vi "Test_PicoScope_v2.vi"() -> ()   [LabVIEW 2015]
uses:
  Controls/PicoScope/pico_control_panel.ctl
  Controls/PicoScope/pico_channel_settings.ctl
  Controls/PicoScope/pico_trigger.ctl
  Controls/PicoScope/pico_init_settings.ctl
panel:
  out "Pico Scope Channel B":T1(graph)
  out "Pico Scope Channel A":T1(graph)
  in  "error in (no error)":errorcluster
  out "error out":errorcluster
  in  "PicoScope Acquisition Settings Input":T2={"Channel A Settings"={"Enabled"=TRUE, "Coupling"=1, "Range"=6, "Analogue Offset"=0.0}, "Channel B Settings"={"Enabled"=TRUE, "Coupling"=1, "Range"=6, "Analogue Offset"=0.0}, "Trigger Options"={"Trigger Enabled"=FALSE, "Trigger Source"=enum."Channel A", "Trigger Threshold (-5 to 5 V)"=0.0, "Trigger Slope"=2, "Trigger Delay (ms)"=0.0, "Auto Trigger Time (ms)"=1000}, "Pico Scope Inititalization Settings"={"USB Power"=FALSE, "Use Serial Number"=FALSE, "Resolution"=0, "Serial Number"="", "Handle"=0}, "Use PicoScope?"=FALSE, "Acquisition Settings"={"Pre Trigger Time (s)"=512.0, "Post Trigger Time (s)"=512.0, "Resolution (s)"=34.36, "Four Channel Device"=FALSE, "Number of Captures"=1.0}} {"Acquisition Settings"."Number of Captures" min=1.0 step=1.0; "Acquisition Settings"."Resolution (s)" min=1e-09 max=34.36 step=1e-09 format="%#_6p"; "Acquisition Settings"."Post Trigger Time (s)" min=0.0 format="%#_6p"; "Acquisition Settings"."Pre Trigger Time (s)" min=0.0 format="%#_6p"; "Pico Scope Inititalization Settings"."Resolution" items=["8-bit", "12-bit", "14-bit", "15-bit (max. 2 ch.)", "16-bit (max. 1 ch.)"]; "Trigger Options"."Trigger Slope" items=["Rising"=2, "Falling"=3]; "Channel B Settings"."Range" items=["10 mV", "20 mV", "50 mV", "100 mV", "200 mV", "500 mV", "1 V", "2 V", "5 V", "10 V", "20 V", "50 V ", "100 V"]; "Channel B Settings"."Coupling" items=["AC", "DC"]; "Channel A Settings"."Range" items=["10 mV", "20 mV", "50 mV", "100 mV", "200 mV", "500 mV", "1 V", "2 V", "5 V", "10 V", "20 V", "50 V ", "100 V"]; "Channel A Settings"."Coupling" items=["AC", "DC"]}
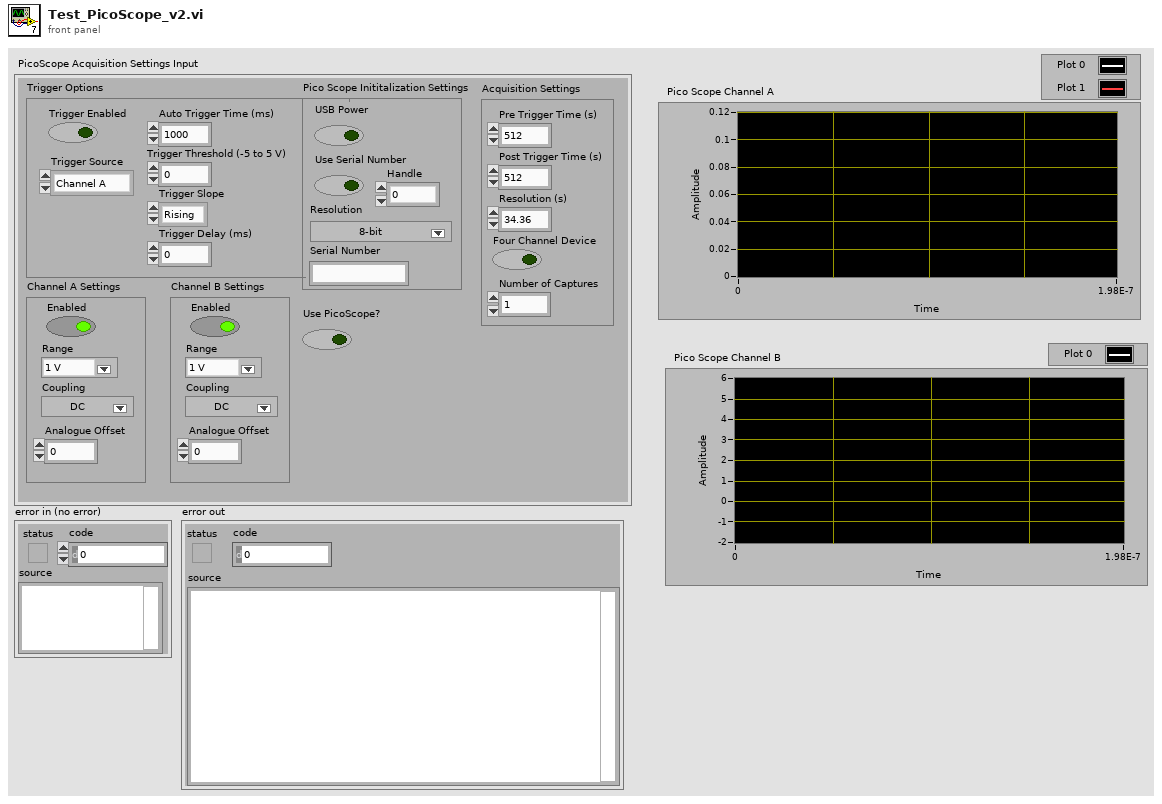
[diagram p1: front panel]
types:
  T1 = cluster{"Channel A Out":dbl[], "Channel A Out":dbl[]}[]
  T2 = typedef "pico_control_panel.ctl" = cluster{"Channel A Settings":T3, "Channel B Settings":T3, "Trigger Options":T4, "Pico Scope Inititalization Settings":T5, "Use PicoScope?":bool, "Acquisition Settings":cluster{"Pre Trigger Time (s)":dbl, "Post Trigger Time (s)":dbl, "Resolution (s)":dbl, "Four Channel Device":bool, "Number of Captures":dbl}}
  T3 = typedef "pico_channel_settings.ctl" = cluster{"Enabled":bool, "Coupling":i16, "Range":u16, "Analogue Offset":sgl}
  T4 = typedef "pico_trigger.ctl" = cluster{"Trigger Enabled":bool, "Trigger Source":enum16{"Channel A", "Channel B", "Channel C", "Channel D", "Ext."}, "Trigger Threshold (-5 to 5 V)":dbl, "Trigger Slope":u16, "Trigger Delay (ms)":dbl, "Auto Trigger Time (ms)":i16}
  T5 = typedef "pico_init_settings.ctl" = cluster{"USB Power":bool, "Use Serial Number":bool, "Resolution":i32, "Serial Number":string, "Handle":i16}
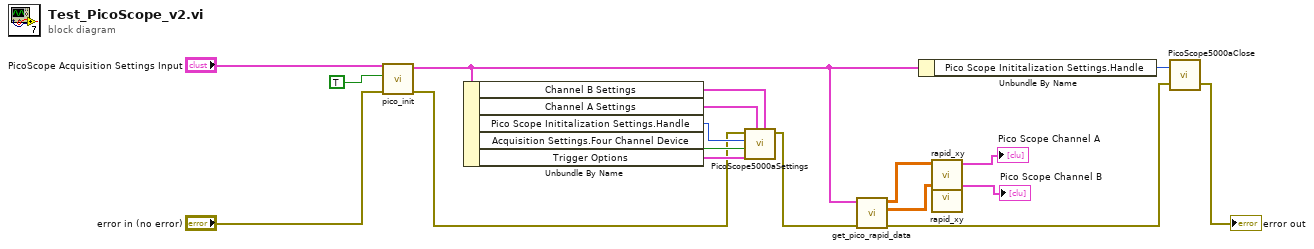
[diagram p0: block diagram]
diagram:
  n1 = call "pico_init.vi"("error in (no error)"="error in (no error)", "Initialize PicoScope?"=TRUE, "PicoScope Acquisition Settings Input"="PicoScope Acquisition Settings Input") -> ("error out"=w7:errorcluster, "PicoScope Acquisition Settings Output"=w5:T2)  [unwired: 4 in, 2 out]
  n2 = Unbundle By Name(w5) -> ("Channel B Settings"=w12:T3, "Channel A Settings"=w11:T3, "Pico Scope Inititalization Settings.Handle"=w10:i16, "Acquisition Settings.Four Channel Device"=w9:bool, "Trigger Options"=w8:T4)
  n3 = call "PicoScope5000aSettings.vi"("Channel B Settings"=w12, "Channel A Settings"=w11, "Trigger Settings"=w8, "Four Channel Device?"=w9, "handle in"=w10, "error in"=w7) -> ("error out"=w6:errorcluster)  [unwired: 4 in, 1 out]
  n4 = call "get_pico_rapid_data.vi"("error in"=w6, "PicoScope Acquisition Settings"=w5) -> ("error out"=w17:errorcluster, "Channel B Out"=w1:dbl[][][], "Channel A Out"=w4:dbl[][][])  [unwired: 7 in]
  n5 = Unbundle By Name(w5) -> ("Pico Scope Inititalization Settings.Handle"=w14:i16)
  n6 = call "rapid_xy.vi"("Channel A Out"=w4) -> ("xy array"=→"Pico Scope Channel A":T1)  [unwired: 10 in]
  n7 = call "rapid_xy.vi"("Channel A Out"=w1) -> ("xy array"=→"Pico Scope Channel B":T1)  [unwired: 10 in]
  n8 = call "PicoScope5000aClose.vi"("error in (no error)"=w17, "handle"=w14) -> ("error out"=→"error out":errorcluster)  [unwired: 1 in]
